vi "GetStatusInfo.vi"(4 "error in":errorcluster, 5 "Camera In":T2) -> (0 "Status Info":T1, 1 "error out":errorcluster, 2 "Camera Out":T2)   [LabVIEW 2013]
uses:
  <vilib>/userdefined/High Color/IMAQdx.ctl
  <resource>/objmgr/imaqdx.rc
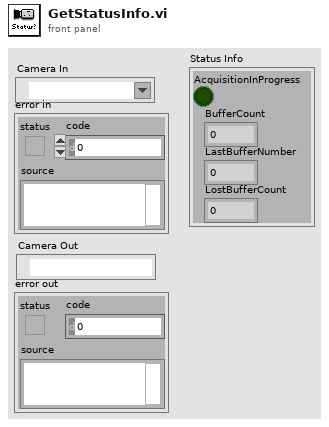
[diagram p1: front panel]
types:
  T1 = cluster{"AcquisitionInProgress":bool, "BufferCount":u32, "LastBufferNumber":u32, "LostBufferCount":u32}
  T2 = typedef "IMAQdx.ctl" = refnum<k21>
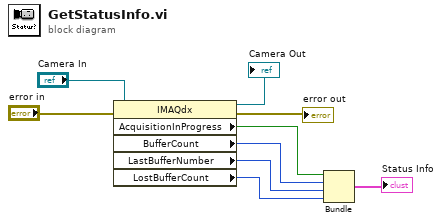
[diagram p0: block diagram]
diagram:
  n1 = property class="IMAQdx"(reference="Camera In", error in="error in") -> (reference out=→"Camera Out":T2, error out=→"error out":errorcluster, "AcquisitionInProgress"=w5:bool, "BufferCount"=w2:u32, "LastBufferNumber"=w3:u32, "LostBufferCount"=w4:u32)
  n2 = Bundle("AcquisitionInProgress"=w5, "BufferCount"=w2, "LastBufferNumber"=w3, "LostBufferCount"=w4) -> (→"Status Info":T1)  [unwired: 1 in]
